vi "Core_Host.vi"() -> ()   [LabVIEW 2017]
uses:
  <vilib>/Utility/file.llb/Read Delimited Spreadsheet (DBL).vi
panel:
  in  "Dyn. Power Profile File":path
  in  "Load Power Profile":bool
  in  "stop":bool
  out "Profile Step":i32
  out "Power Output":dbl
  out "Power Input Signal":dbl
  out "Output Current 2":dbl
  out "Output Voltage 2":dbl
  out "Output Current 1":dbl
  out "Output Voltage 1":dbl
  out "Loop Period":i64
  in  "Shutdown":bool
  in  "Desired Power":dbl
  in  "Select Operation Mode":u16
  in  "Power Output On":bool
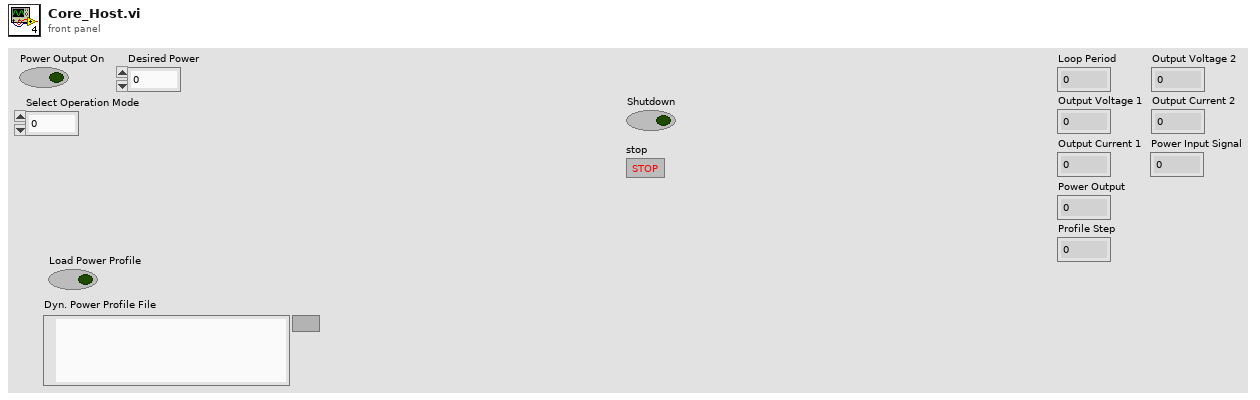
[diagram p1: front panel]
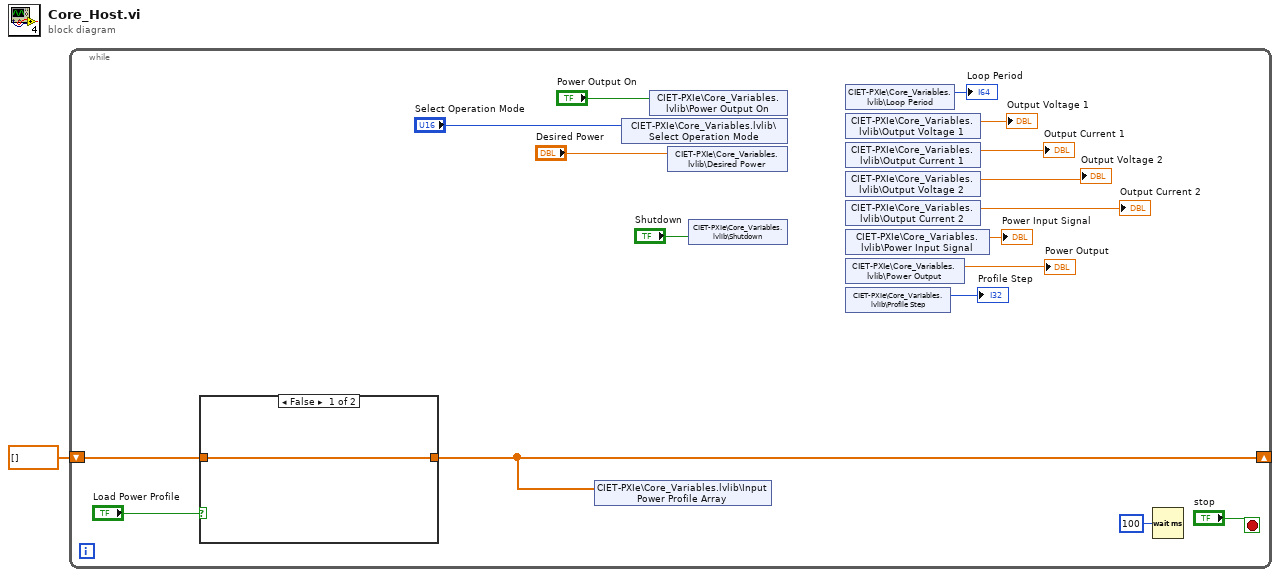
[diagram p0: block diagram]
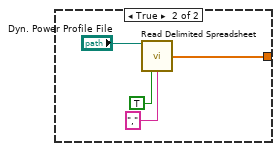
[diagram p2: hidden frame]
diagram:
  n1 = while {
    shift-right: [w2] -> _
    shift-left: dbl[] [] ("Input Power Profile Array") -> [w3]
    stop <- "stop" stop-if-true
    n2 = case shown="False" "Load Power Profile" {
      tunnel: [w19 w20] -> w2
      tunnel: w3 -> [w19 _]
      frame False {
      }
      frame True {
        n3 = call-poly <vilib>:"Read Delimited Spreadsheet.vi"("file path (dialog if empty)"="Dyn. Power Profile File", "transpose? (F)"=TRUE, "delimiter (\\t)"="," ("delimiter (\\t)")) -> ("first row"=w20:dbl[])  [unwired: 7 in, 5 out]
      }
    }
    n4 = shared-variable "CIET-PXIe\\Core_Variables.lvlib\\Input Power Profile Array"(w2) -> ()  [unwired: 1 in, 1 out]
    n5 = shared-variable "CIET-PXIe\\Core_Variables.lvlib\\Select Operation Mode"("Select Operation Mode") -> ()  [unwired: 1 in, 1 out]
    n6 = shared-variable "CIET-PXIe\\Core_Variables.lvlib\\Power Output On"("Power Output On") -> ()  [unwired: 1 in, 1 out]
    n7 = shared-variable "CIET-PXIe\\Core_Variables.lvlib\\Desired Power"("Desired Power") -> ()  [unwired: 1 in, 1 out]
    n8 = shared-variable "CIET-PXIe\\Core_Variables.lvlib\\Shutdown"("Shutdown") -> ()  [unwired: 1 in, 1 out]
    n9 = shared-variable "CIET-PXIe\\Core_Variables.lvlib\\Loop Period"() -> (→"Loop Period":i64)  [unwired: 1 in, 1 out]
    n10 = shared-variable "CIET-PXIe\\Core_Variables.lvlib\\Output Voltage 1"() -> (→"Output Voltage 1":dbl)  [unwired: 1 in, 1 out]
    n11 = shared-variable "CIET-PXIe\\Core_Variables.lvlib\\Output Current 1"() -> (→"Output Current 1":dbl)  [unwired: 1 in, 1 out]
    n12 = shared-variable "CIET-PXIe\\Core_Variables.lvlib\\Output Voltage 2"() -> (→"Output Voltage 2":dbl)  [unwired: 1 in, 1 out]
    n13 = shared-variable "CIET-PXIe\\Core_Variables.lvlib\\Output Current 2"() -> (→"Output Current 2":dbl)  [unwired: 1 in, 1 out]
    n14 = shared-variable "CIET-PXIe\\Core_Variables.lvlib\\Power Input Signal"() -> (→"Power Input Signal":dbl)  [unwired: 1 in, 1 out]
    n15 = shared-variable "CIET-PXIe\\Core_Variables.lvlib\\Power Output"() -> (→"Power Output":dbl)  [unwired: 1 in, 1 out]
    n16 = shared-variable "CIET-PXIe\\Core_Variables.lvlib\\Profile Step"() -> (→"Profile Step":i32)  [unwired: 1 in, 1 out]
    n17 = Wait (ms)(milliseconds to wait=u32 100) -> ()  [unwired: 1 out]
  }
